vi "process controller save method.vi"(6 "default or user":T1, 8 "error in (not an error)":errorcluster, 9 "TCP ID":refnum<k5>, 10 "Action":T5, 11 "Plant method in":T3={"Operator information"=[], "data log interval"=60, "data loop interval"=10, "Datalog directory path"=path "", "graph update interval"=1.0, "history length"=1000, "Control Logic file path"=path "", "Sensor Configuration file path"=path "", "HMI VI path"=path "", "HMI data smooth"=5.0} {"HMI data smooth" min=0.01 format="%.2f"; "history length" min=1; "graph update interval" min=0.1 format="%.2f"; "data log interval" min=1}) -> (0 "error out":errorcluster, 1 "sensor &var names":string[](array[string]), 2 "State names":string[](array[string]), 3 "Plant method out":T3={"Operator information"=[], "data log interval"=60, "data loop interval"=10, "Datalog directory path"=path "", "graph update interval"=1.0, "history length"=1000, "Control Logic file path"=path "", "Sensor Configuration file path"=path "", "HMI VI path"=path "", "HMI data smooth"=5.0} {"HMI data smooth" min=0.01 format="%.2f"; "history length" min=1; "graph update interval" min=0.1 format="%.2f"; "data log interval" min=1}, 5 "output descriptions out":string[][](array[string]))   [LabVIEW 2012]
uses:
  file/file action.ctl
  Plant method.ctl
  operator info.ctl
  DAQ configuration/channel identifierbc1.ctl
  default or user select.ctl
  logic buffer cmd.ctl
  DAC project/Calibration and Function folders.ctl
  calibration/global scale array.vi
panel:
  in  "sensor array bc1":T2[](array[typedef]) {"channel" max=31; "module" min=1 step=1}
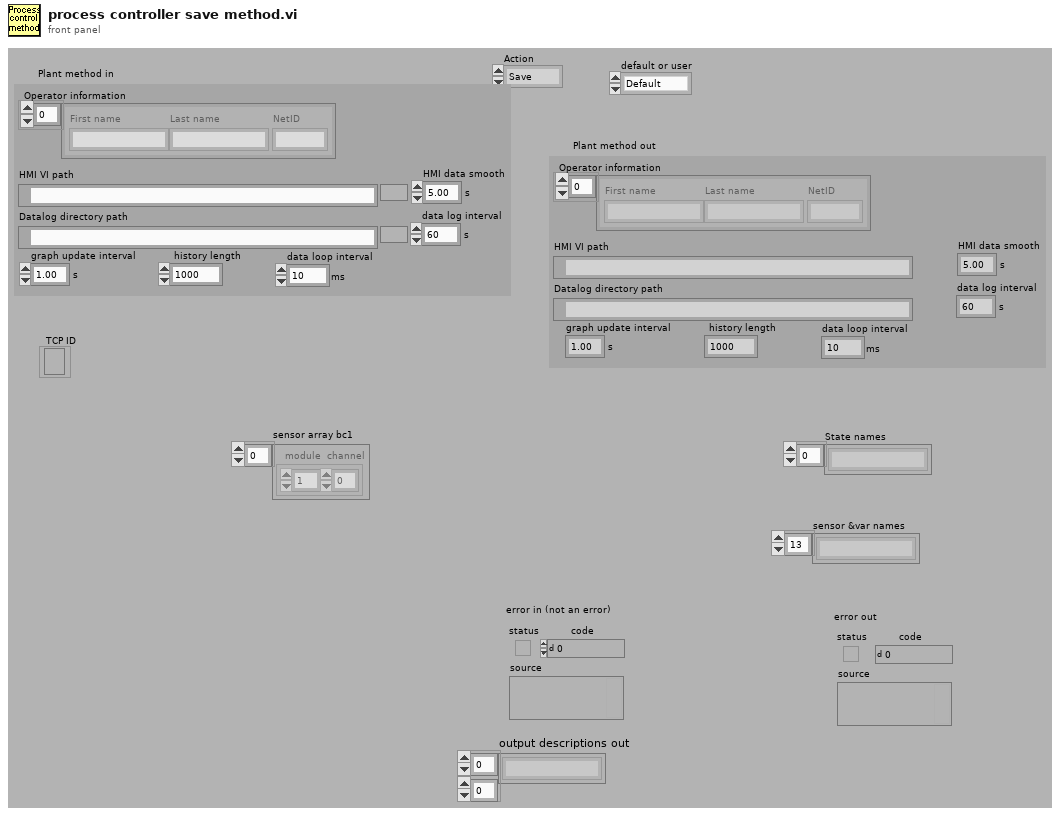
[diagram p1: front panel]
types:
  T1 = typedef "default or user select.ctl" = enum16{"Default", "User select"}
  T2 = typedef "channel identifierbc1.ctl" = cluster{"module":u8, "channel":u8}
  T3 = typedef "Plant method.ctl" = cluster{"Operator information":T4, "data log interval":u32, "data loop interval":u32, "Datalog directory path":path, "graph update interval":sgl, "history length":u16, "Control Logic file path":path, "Sensor Configuration file path":path, "HMI VI path":path, "HMI data smooth":dbl}
  T4 = typedef "operator info.ctl" = cluster{"First name":string, "Last name":string, "NetID":string}[]
  T5 = typedef "file action.ctl" = enum16{"Save", "Open"}
  T6 = typedef "logic buffer cmd.ctl" = enum16{"read", "write ouput settings", "write rules", "write setpoints", "write output descriptions", "write all", "calculate setpoints", "save", "open", "Load all setpoint code", "Load one setpoint code", "Configure one setpoint code"}
  T7 = typedef "calib array.ctl" = T8[]
  T8 = typedef "conversion.ctl" = cluster{"conversion matrix":sgl[][], "units":string, "name":string, "scale type":T9, "offset (volts)":dbl, "second channel":i8, "correspondence table":T10, "offset (physical units)":dbl, "pH scale":T11, "D.O.":T12}
  T9 = typedef "scale type.ctl" = enum16{"Volts", "Polynomial", "Correspondence Table", "pH", "Dissolved Oxygen", "Quadratic"}
  T10 = typedef "correspondence table.ctl" = cluster{"physical units":dbl, "volts":dbl}[]
  T11 = typedef "pH scale.ctl" = cluster{"Buffers":cluster{"Buffer":dbl, "Calibrated":bool, "V/T":dbl}[], "Temperature":dbl}
  T12 = typedef "DO scale.ctl" = cluster{"Temperature":dbl, "K":dbl, "barometric pressure":dbl}
  T13 = typedef "Sensor array.ctl" = T14[]
  T14 = typedef "channel identifier.ctl" = u16
  T15 = typedef "variable setpoint.ctl" = cluster{"name":string, "unit":string, "value":dbl, "Type":enum16{"Constant", "Variable"}, "variable":cluster{"selected sensors":i32[], "selected set points":i32[], "VI":path, "Data average interval":T16, "code ref":T17}}
  T16 = typedef "data ave interval.ctl" = dbl
  T17 = typedef "type specifier for control code.ctl" = refnum<vi>
  T18 = typedef "Output control.ctl" = u16[][]
  T19 = typedef "rules.ctl" = T20[]
  T20 = typedef "State rules.ctl" = cluster{"state rules":T21[], "State name":string}
  T21 = typedef "rule.ctl" = cluster{"next state":u16, "conditions":T22[], "number of conditions":u8, "Rule name":string}
  T22 = typedef "condition.ctl" = cluster{"> or <":T23, "set point":i32, "sensors and variables":i32, "Data average interval":dbl}
  T23 = typedef "greater or less.ctl" = bool
  T24 = cluster{"Plant method in":T3, "Calibration matrix":T7, "Sensor Array out":T13, "Set Points out":T15[], "ouput settings out":T18, "Rules out":T19, "output descriptions out":string[][]}
  T25 = typedef "Calibration and Function folders.ctl" = enum16{"Sensors", "Functions", "Config File", "UserAppFolder"}
  T26 = cluster{"Plant method in":T3, "Calibration matrix":T7, "sensor array bc1":T2[], "Set Points out":T15[], "ouput settings out":T18, "Rules out":T19, "output descriptions out":string[][]}
  T27 = cluster{"Plant method in":T3, "Calibration matrix":T7, "Channel Indices":i32[], "Set Points out":T15[], "ouput settings out":T18, "Rules out":T19, "output descriptions out":string[][]}
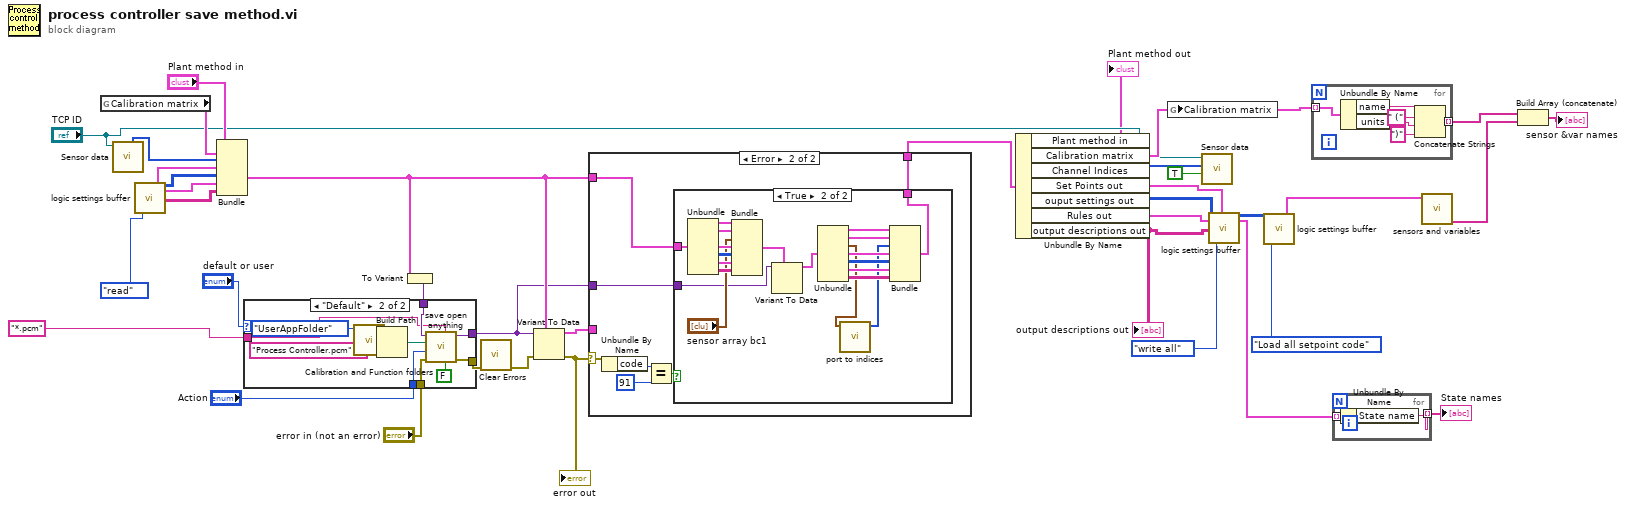
[diagram p0: block diagram]
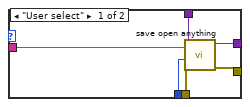
[diagram p2: hidden frame]
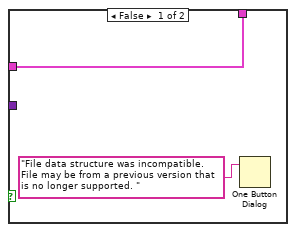
[diagram p4: hidden frame]
diagram:
  n1 = global read "global scale array.vi" "Calibration matrix"() -> (w37:T7)
  n2 = call "Sensor data.vi"("Connection ID in"="TCP ID") -> ("Sensor Array out"=w30:T13)  [unwired: 3 in, 7 out]
  n3 = call "logic settings buffer.vi"("command"=logic_buffer_cmd."read") -> ("Set Points out"=w10:T15[], "ouput settings out"=w29:T18, "Rules out"=w28:T19, "output descriptions out"=w18:string[][])  [unwired: 11 in, 4 out]
  n4 = Bundle("Plant method in"="Plant method in", "Calibration matrix"=w37, "Sensor Array out"=w30, "Set Points out"=w10, "ouput settings out"=w29, "Rules out"=w28, "output descriptions out"=w18) -> (w5:T24)  [unwired: 1 in]
  n5 = To Variant(anything=w5) -> (Variant=w35:variant)
  n6 = case shown="\"Default\"" "default or user" {
    tunnel: "Action" -> [w44 w51]
    tunnel: w35 -> [w43 w53]
    tunnel: "error in (not an error)" -> [w42 w52]
    tunnel: [w41 w54] -> w32
    tunnel: "*.pcm" ("pattern") -> [w39 w48]
    tunnel: [w40 w55] -> w4
    frame "User select" {
      n7 = call "save open anything.vi"("Variant"=w43, "Action"=w44, "error in (not an error)"=w42, "pattern"=w39) -> ("Variant out"=w40:variant, "error out"=w41:errorcluster)  [unwired: 3 in, 2 out]
    }
    frame "Default" {
      n8 = call "Calibration and Function folders.vi"("Folder"=Calibration_and_Function_folders."UserAppFolder") -> ("Selected Folder"=w45:path)  [unwired: 10 in]
      n9 = Build Path(base path=w45, name or relative path="Process Controller.pcm") -> (appended path=w49:path)
      n10 = call "save open anything.vi"("Variant"=w53, "file path"=w49, "Action"=w51, "error in (not an error)"=w52, "pattern"=w48, "advisory dialog? (display:T)"=FALSE) -> ("Variant out"=w55:variant, "error out"=w54:errorcluster)  [unwired: 1 in, 2 out]
    }
  }
  n11 = call <vilib>:"Clear Errors.vi"("error in (no error)"=w32) -> ("error out"=w31:errorcluster)  [unwired: 6 in]
  n12 = Variant To Data(error in=w31, type=w5, Variant=w4) -> (data=w12:T24, error out=w14:errorcluster)
  "error out" <- w14
  n13 = case shown="Error" w14 {
    selector: w14 -> [_ w63]
    tunnel: [w56 w57] -> w13
    tunnel: w5 -> [_ w59]
    tunnel: w12 -> [w56 _]
    tunnel: w4 -> [_ w58]
    frame No Error {
    }
    frame Error {
      n14 = Unbundle By Name(w63) -> ("code"=w62:i32)
      n15 = Equal?(x=w62, y=91) -> (x = y?=w60:bool)
      n16 = case shown="True" w60 {
        tunnel: w59 -> [w64 w85]
        tunnel: w58 -> [_ w76]
        tunnel: [w64 w66] -> w57
        frame False {
          n17 = One Button Dialog(message="File data structure was incompatible. File may be from a previous version that is no longer supported. ") -> ()  [unwired: 1 in, 1 out]
        }
        frame True {
          n18 = Unbundle(w85) -> ("Plant method in"=w84:T3, "Calibration matrix"=w83:T7, "Set Points out"=w82:T15[], "ouput settings out"=w81:T18, "Rules out"=w80:T19, "output descriptions out"=w79:string[][])  [unwired: 1 out]
          n19 = Bundle("Plant method in"=w84, "Calibration matrix"=w83, "sensor array bc1"="sensor array bc1", "Set Points out"=w82, "ouput settings out"=w81, "Rules out"=w80, "output descriptions out"=w79) -> (w77:T26)  [unwired: 1 in]
          n20 = Variant To Data(type=w77, Variant=w76) -> (data=w71:T26)  [unwired: 1 in, 1 out]
          n21 = Unbundle(w71) -> ("Plant method in"=w72:T3, "Calibration matrix"=w73:T7, "sensor array bc1"=w68:T2[], "Set Points out"=w74:T15[], "ouput settings out"=w75:T18, "Rules out"=w69:T19, "output descriptions out"=w70:string[][])
          n22 = call "port to indices.vi"("Port"=w68) -> ("Channel Indices"=w67:i32[])  [unwired: 10 in]
          n23 = Bundle("Plant method in"=w72, "Calibration matrix"=w73, "Channel Indices"=w67, "Set Points out"=w74, "ouput settings out"=w75, "Rules out"=w69, "output descriptions out"=w70) -> (w66:T27)  [unwired: 1 in]
        }
      }
    }
  }
  n24 = Unbundle By Name(w13) -> ("Plant method in"=→"Plant method out":T3, "Calibration matrix"=w33:T7, "Channel Indices"=w27:i32[], "Set Points out"=w2:T15[], "ouput settings out"=w25:T18, "Rules out"=w24:T19, "output descriptions out"=w17:string[][])
  "output descriptions out" <- w17
  n25 = global write "global scale array.vi" "Calibration matrix"(w33) -> ()
  n26 = call "Sensor data.vi"("Update channels"=TRUE, "Sensor Array"=w27, "Connection ID in"="TCP ID") -> ()  [unwired: 1 in, 8 out]
  n27 = call "logic settings buffer.vi"("output settings"=w25, "Rules"=w24, "output descriptions"=w17, "command"=logic_buffer_cmd."write all", "Set Points"=w2) -> ("ouput settings out"=w16:T18, "Rules out"=w23:T19)  [unwired: 7 in, 6 out]
  n28 = call "logic settings buffer.vi"("output settings"=w16, "command"=logic_buffer_cmd."Load all setpoint code") -> ("Set Points out"=w6:T15[])  [unwired: 10 in, 7 out]
  n29 = for {
    tunnel: w33 -> [w91] mode=indexing
    tunnel: [w86] -> w8 mode=indexing
    n30 = Unbundle By Name(w91) -> ("name"=w90:string, "units"=w88:string)
    n31 = Concatenate Strings(w90, " (" ("string"), w88, ")" ("string")) -> (w86:string)
  }
  n32 = for {
    tunnel: w23 -> [w93] mode=indexing
    tunnel: [w92] -> w22 mode=indexing
    n33 = Unbundle By Name(w93) -> ("State name"=w92:string)
  }
  "State names" <- w22
  n34 = call "sensors and variables.vi"("S P & V definitions"=w6) -> ("name (unit)"=w9:string[])  [unwired: 7 in, 3 out]
  n35 = Build Array (concatenate)(w8, w9) -> (→"sensor &var names":string[])
